vi "Get Schema Version.vi"(8 "error in":errorcluster, 11 "Configuration file in":path) -> (0 "error out":errorcluster, 2 "schema version":string, 3 "Configuration file out":path)   [LabVIEW 2020]
uses:
  <vilib>/xml/NI_XML.lvlib
  <vilib>/xml/Close Reference(Node).vi
  <resource>/objmgr/DOMUserDefRef.rc
  <vilib>/xml/Close Reference(NNMap).vi
  <vilib>/xml/Load XML File.vi
  <vilib>/xml/Close Reference(NdList).vi
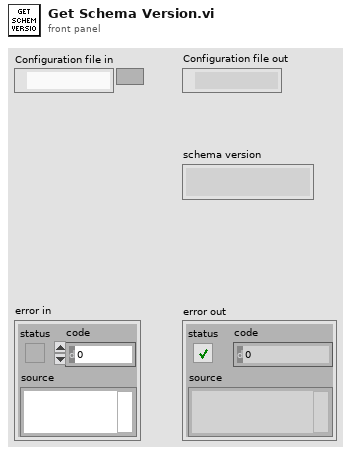
[diagram p1: front panel]
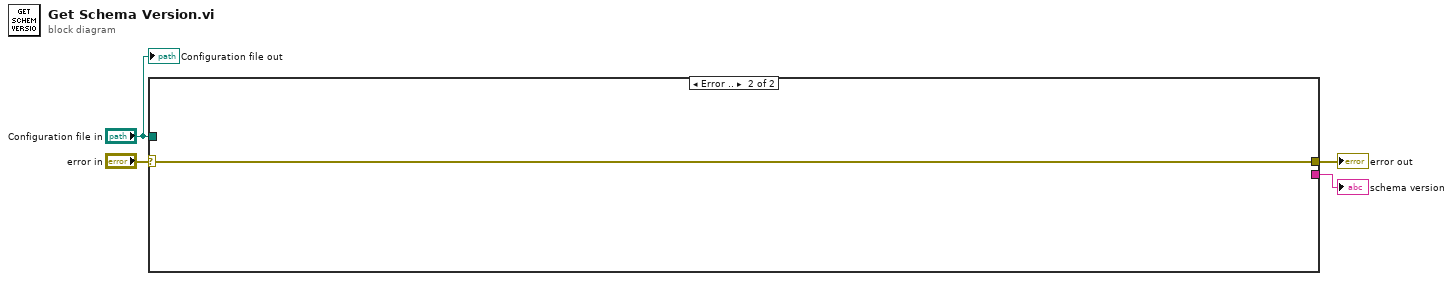
[diagram p0: block diagram]
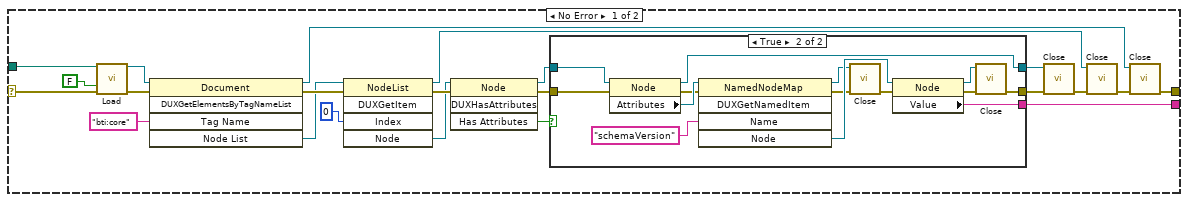
[diagram p2: hidden frame]
diagram:
  n1 = case shown="Error .." "error in" {
    selector: "error in" -> [w5 w43]
    tunnel: [w21 _] -> w4
    tunnel: [w11 w43] -> w3
    tunnel: "Configuration file in" -> [w8 _]
    frame No Error {
      n2 = call-poly <vilib>:"Load.vi"("path to XML document"=w8, "load external DTD (True)"=FALSE, "error in (no error)"=w5) -> ("DOM document out"=w6:refnum<k20>, "error out"=w7:errorcluster)  [unwired: 10 in, 1 out]
      n3 = invoke class="Document" method="DUXGetElementsByTagNameList"(reference=w6, error in=w7, "Tag Name"="bti:core") -> (reference out=w9:refnum<k20>, error out=w15:errorcluster, "Node List"=w13:refnum<k20>)  [unwired: 2 in, 2 out]
      n4 = invoke class="NodeList" method="DUXGetItem"(reference=w13, error in=w15, "Index"=0) -> (reference out=w26:refnum<k20>, error out=w17:errorcluster, "Node"=w16:refnum<k20>)  [unwired: 2 in, 2 out]
      n5 = invoke class="Node" method="DUXHasAttributes"(reference=w16, error in=w17) -> (reference out=w20:refnum<k20>, error out=w19:errorcluster, "Has Attributes"=w18:bool)  [unwired: 2 in, 1 out]
      n6 = case shown="True" w18 {
        tunnel: w19 -> [w27 w41]
        tunnel: w20 -> [w28 w42]
        tunnel: [_ w37] -> w21
        tunnel: [w28 w31] -> w22
        tunnel: [w27 w29] -> w23
        frame False {
        }
        frame True {
          n7 = property class="Node"(reference=w42, error in=w41) -> (reference out=w31:refnum<k20>, error out=w30:errorcluster, "Attributes"=w40:refnum<k20>)
          n8 = invoke class="NamedNodeMap" method="DUXGetNamedItem"(reference=w40, error in=w30, "Name"="schemaVersion") -> (reference out=w33:refnum<k20>, error out=w34:errorcluster, "Node"=w38:refnum<k20>)  [unwired: 2 in, 2 out]
          n9 = call-poly <vilib>:"Close.vi"("error in (no error)"=w34, "named node map"=w33) -> ("error out"=w32:errorcluster)  [unwired: 7 in]
          n10 = property class="Node"(reference=w38, error in=w32) -> (reference out=w35:refnum<k20>, error out=w36:errorcluster, "Value"=w37:string)
          n11 = call-poly <vilib>:"Close.vi"("error in (no error)"=w36, "node"=w35) -> ("error out"=w29:errorcluster)  [unwired: 7 in]
        }
      }
      n12 = call-poly <vilib>:"Close.vi"("error in (no error)"=w23, "node"=w22) -> ("error out"=w24:errorcluster)  [unwired: 7 in]
      n13 = call-poly <vilib>:"Close.vi"("error in (no error)"=w24, "node list"=w26) -> ("error out"=w25:errorcluster)  [unwired: 7 in]
      n14 = call-poly <vilib>:"Close.vi"("error in (no error)"=w25, "node"=w9) -> ("error out"=w11:errorcluster)  [unwired: 7 in]
    }
    frame Error {
    }
  }
  "schema version" <- w4
  "error out" <- w3
  "Configuration file out" <- "Configuration file in"
